vi "APU Simulation Test.vi"() -> ()   [LabVIEW 2015]
uses:
  IP Source/APU/Settings.ctl
  IP Source/APU/APU.lvlib
  IP Source/APU/Input.ctl
  IP Source/APU/Register Bus.ctl
  IP Source/APU/Shared Settings.ctl
panel:
  in  "enable accel":bool
  in  "IP to use":enum16{"Old APU", "New APU"}(ring)
  out "Speed Error (%)":dbl=3.708733452185698e-05
  out "Actual Speed":dbl=6000.002225240071 format="%#_15g"
  out "Acceleration Error (%)":dbl=nan
  out "Actual acceleration":dbl=993408.8514758819
  out "Actual Speed":dbl[](graph)
  in  "Desired Speed (RPM)":dbl=6000.0 format="%#_13g"
  out "Cycle":dbl[](graph)
  out "Crank":dbl[](graph)
  in  "acceleration (RPM/sec)":dbl=inf
  in  "Crank Revolutions":dbl=4.0 format="%#_15g"
  # "ONLY WORKS FOR NEW IP"
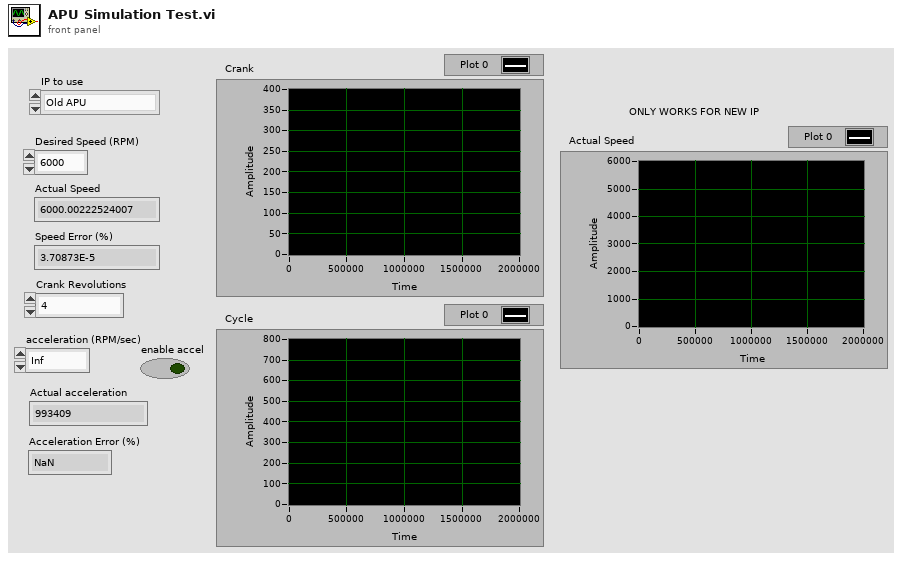
[diagram p1: front panel]
types:
  T1 = typedef "Engine Simulation Toolkit.lvlib/APU.lvlib/Settings.ctl" = cluster{"acceleration":fxp<+,18,-20>, "enable accel":bool}
  T2 = typedef "Engine Simulation Toolkit.lvlib/APU.lvlib/Register Bus.ctl" = cluster{"Speed":refnum<k21>, "Crank Angle":refnum<k21>, "Cycle Angle":refnum<k21>, "Crank Count":refnum<k21>, "Cycle Count":refnum<k21>, "1.25 MHz Counter":refnum<k21>, "Crank Rollover":refnum<k21>, "Cycle Rollover":refnum<k21>, "shared settings":T3}
  T3 = typedef "Engine Simulation Toolkit.lvlib/APU.lvlib/Shared Settings.ctl" = cluster{"start":fxp<+,17,17>, "stuck limit":fxp<+,18,18>}
  T4 = typedef "Engine Simulation Toolkit.lvlib/APU.lvlib/Input.ctl" = cluster{"desired speed":fxp<+/-,23,2>, "reset":bool}
  T5 = typedef "Engine Simulation Toolkit.lvlib/APU.lvlib/Output.ctl" = cluster{"crank":u16, "cycle":u16, "actual speed":fxp<+/-,23,2>}
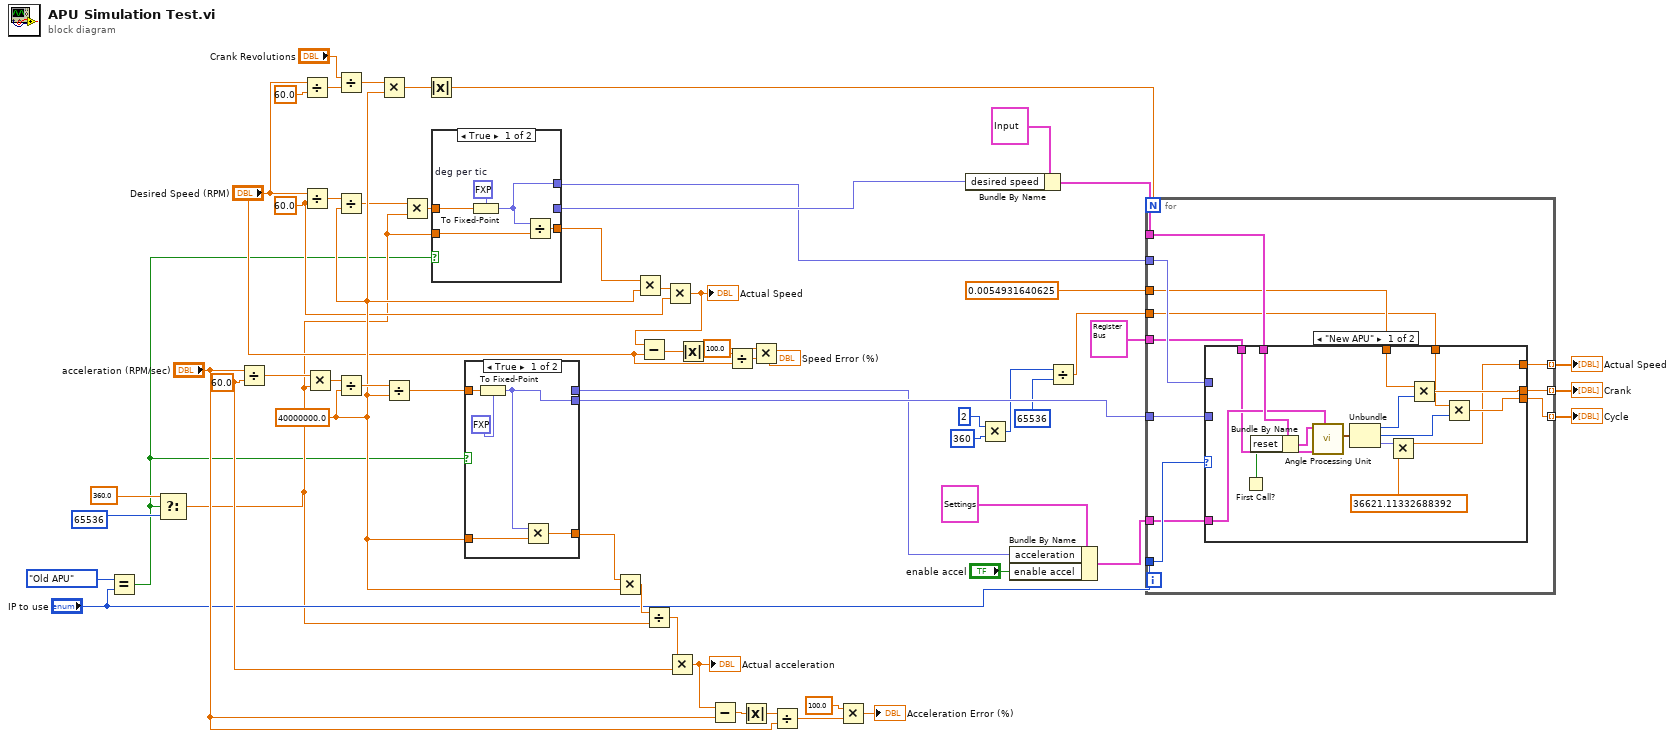
[diagram p0: block diagram]
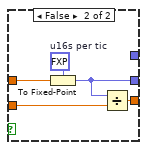
[diagram p2: hidden frame]
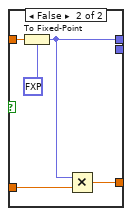
[diagram p3: hidden frame]
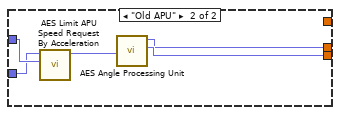
[diagram p4: hidden frame]
diagram:
  w44 = 60.0 ("y")
  w33 = 60.0 ("y")
  w35 = 40000000.0 ("y")
  n1 = Equal?(x=enum16{"Old APU", "Rate Limited APU", "APU"}."Old APU", y="IP to use") -> (x = y?=w10:bool)
  n2 = Select(t=360.0 ("y"), s=w10, f=u32 65536 ("n")) -> (s? t:f=w12:dbl)
  n3 = Divide(x="acceleration (RPM/sec)", y=w44) -> (x/y=w52:dbl)
  n4 = Divide(x="Desired Speed (RPM)", y=60.0) -> (x/y=w56:dbl)
  n5 = Divide(x="Desired Speed (RPM)", y=w33) -> (x/y=w53:dbl)
  n6 = Multiply(x=w52, y=w12) -> (x*y=w51:dbl)
  n7 = Divide(x="Crank Revolutions", y=w56) -> (x/y=w54:dbl)
  n8 = Divide(x=w53, y=w35) -> (x/y=w17:dbl)
  n9 = Divide(x=w51, y=w35) -> (x/y=w50:dbl)
  n10 = Multiply(x=w54, y=w35) -> (x*y=w60:dbl)
  n11 = Divide(x=w50, y=w35) -> (x/y=w48:dbl)
  n12 = Multiply(x=w17, y=w12) -> (x*y=w49:dbl)
  n13 = Absolute Value(x=w60) -> (abs(x)=w25:dbl)
  n14 = case shown="True" w10 {
    tunnel: w49 -> [w65 w70]
    tunnel: [w64 w69] -> w36
    tunnel: [_ w68] -> w23
    tunnel: w12 -> [w62 w66]
    tunnel: [w61 _] -> w9
    frame True {
      w63 = fxp<+/-,47,-4> 0.0  # deg per tic
      n15 = To Fixed-Point(fixed-point type=w63, number=w65) -> (fixed-point=w61:fxp<+/-,47,-4>)
      n16 = Divide(x=w61, y=w62) -> (x/y=w64:dbl)
    }
    frame False {
      w67 = fxp<+/-,23,2> 0.0  # u16s per tic
      n17 = To Fixed-Point(fixed-point type=w67, number=w70) -> (fixed-point=w68:fxp<+/-,23,2>)
      n18 = Divide(x=w68, y=w66) -> (x/y=w69:dbl)
    }
  }
  n19 = case shown="True" w10 {
    tunnel: w48 -> [w75 w80]
    tunnel: [w74 w79] -> w47
    tunnel: w35 -> [w73 w78]
    tunnel: [_ w77] -> w7
    tunnel: [w72 _] -> w11
    frame True {
      n20 = To Fixed-Point(fixed-point type=fxp<+/-,47,-4> 0.0 ("u16s per tic per tic"), number=w75) -> (fixed-point=w72:fxp<+/-,47,-4>)
      n21 = Multiply(x=w72, y=w73) -> (x*y=w74:dbl)
    }
    frame False {
      n22 = To Fixed-Point(fixed-point type=fxp<+,18,-20> 0.0 ("u16s per tic per tic"), number=w80) -> (fixed-point=w77:fxp<+,18,-20>)
      n23 = Multiply(x=w77, y=w78) -> (x*y=w79:dbl)
    }
  }
  n24 = Multiply(x=w47, y=w35) -> (x*y=w46:dbl)
  n25 = Multiply(x=w36, y=w35) -> (x*y=w34:dbl)
  n26 = Divide(x=w46, y=w12) -> (x/y=w45:dbl)
  n27 = Multiply(x=w34, y=w33) -> (x*y=w27:dbl)
  "Actual Speed" <- w27
  n28 = Subtract(x=w27, y="Desired Speed (RPM)") -> (x-y=w28:dbl)
  n29 = Multiply(x=w45, y=w44) -> (x*y=w43:dbl)
  "Actual acceleration" <- w43
  n30 = Absolute Value(x=w28) -> (abs(x)=w29:dbl)
  n31 = Subtract(x=w43, y="acceleration (RPM/sec)") -> (x-y=w42:dbl)
  n32 = Divide(x=w29, y="Desired Speed (RPM)") -> (x/y=w30:dbl)
  n33 = Absolute Value(x=w42) -> (abs(x)=w41:dbl)
  n34 = Multiply(x=100.0, y=w30) -> (x*y=→"Speed Error (%)":dbl)
  n35 = Divide(x=w41, y="acceleration (RPM/sec)") -> (x/y=w39:dbl)
  n36 = Multiply(x=100.0, y=w39) -> (x*y=→"Acceleration Error (%)":dbl)
  n37 = Bundle By Name(cluster=T4 {"desired speed"=0.0, "reset"=FALSE} ("<user name here>"), "desired speed"=w23) -> (w22:T4)
  n38 = Multiply(x=u16 2, y=u16 360) -> (x*y=w3:u16)
  n39 = Bundle By Name(cluster=T1 {"acceleration"=0.0, "enable accel"=FALSE} ("rate limited APU settings v1.0.0"), "acceleration"=w7, "enable accel"="enable accel") -> (w18:T1)
  n40 = Divide(x=w3, y=u32 65536) -> (x/y=w2:dbl)
  n41 = for {
    N: w25 -> [_]
    tunnel: w9 -> [w91]
    tunnel: [w89] -> w59 mode=indexing
    tunnel: [w90] -> w58 mode=indexing
    tunnel: "IP to use" -> [w88]
    tunnel: T2 {"Speed"="", "Crank Angle"="", "Cycle Angle"="", "Crank Count"="", "Cycle Count"="", "1.25 MHz Counter"="", "Crank Rollover"="", "Cycle Rollover"="", "shared settings"={"start"=0.0, "stuck limit"=0.0}} ("register bus") -> [w87]
    tunnel: w22 -> [w86]
    tunnel: [w85] -> w21 mode=indexing
    tunnel: w18 -> [w84]
    tunnel: w11 -> [w83]
    tunnel: 0.0054931640625 ("x") -> [w82]
    tunnel: w2 -> [w81]
    n42 = case shown="\"New APU\"" w88 {
      tunnel: w91 -> [_ w109]
      tunnel: [w99 w111] -> w90
      tunnel: [w100 w110] -> w89
      tunnel: w87 -> [w94 _]
      tunnel: w86 -> [w106 _]
      tunnel: [w97 _] -> w85
      tunnel: w84 -> [w95 _]
      tunnel: w82 -> [w103 _]
      tunnel: w83 -> [_ w107]
      tunnel: w81 -> [w98 _]
      frame "New APU" {
        n43 = First Call?() -> (First Call?: T/F=w92:bool)
        n44 = Bundle By Name(cluster=w106, "reset"=w92) -> (w93:T4)
        n45 = call "Angle Processing Unit.vi"("settings.<user name>"=w95, "register bus"=w94, "input.<user name>"=w93) -> ("output.<user name>"=w105:T5)  [unwired: 8 in]
        n46 = Unbundle(w105) -> ("crank"=w102:u16, "cycle"=w101:u16, "actual speed"=w104:fxp<+/-,23,2>)
        n47 = Multiply(x=w104, y=36621.11332688392) -> (x*y=w97:dbl)
        n48 = Multiply(x=w103, y=w102) -> (x*y=w100:dbl)
        n49 = Multiply(x=w98, y=w101) -> (x*y=w99:dbl)
      }
      frame "Old APU" {
        n50 = call <userlib>:"AES Limit APU Speed Request By Acceleration.vi"("APU.Degrees per Tick in"=w109, "APU.Increment Rate"=w107) -> ("APU.Degrees per Tick out"=w108:fxp<+/-,47,-4>)  [unwired: 9 in]
        n51 = call <userlib>:"AES Angle Processing Unit.vi"("APU.Degrees per Tick"=w108) -> ("APU.Cycle Angle"=w111:fxp<+,61,10>, "APU.Crank Angle"=w110:fxp<+,60,9>)  [unwired: 9 in]
      }
    }
  }
  "Crank" <- w59
  "Cycle" <- w58
  "Actual Speed" <- w21
